vi "Create from SSH.vi"(8 "Error In":errorcluster, 11 "SSH":refnum<class "SSH.lvclass">) -> (0 "Error Out":errorcluster, 3 "Identity":refnum<class "Agent Identity.lvclass">)   [LabVIEW 2018, in "Toolkit.lvlib" / "Agent Identity.lvclass"]
uses:
  Agent Identity.lvclass
  SSH/SSH.lvclass
  SSH/SSH.lvclass/SSH.ctl
  Agent Identity.lvclass/Agent Identity.ctl
  Toolkit.lvlib
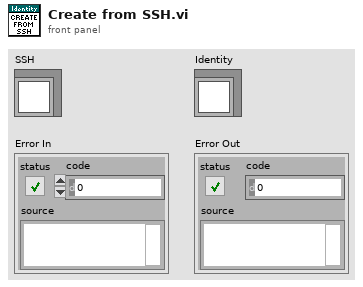
[diagram p1: front panel]
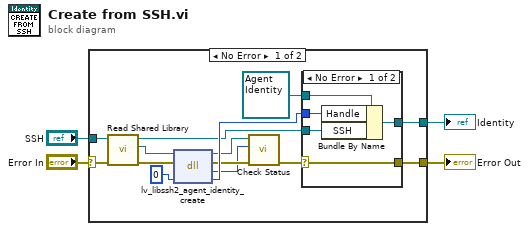
[diagram p0: block diagram]
diagram:
  n1 = case shown="No Error" "Error In" {
    selector: "Error In" -> [w6 w26]
    tunnel: [w9 w26] -> w3
    tunnel: "SSH" -> [w7 _]
    tunnel: [w18 _] -> w1
    frame No Error {
      n2 = call "Read Shared Library.vi"("Error In"=w6, "SSH In"=w7) -> ("Error Out"=w17:errorcluster, "lv-libssh2 Shared Library"=w16:path, "SSH Out"=w8:refnum<class "SSH.lvclass">)  [unwired: 7 in]
      n3 = dll-call lib="libssh2lv.*" fn="lv_libssh2_agent_identity_create"(path in=w16, error in=w17, "handle"=u64 0) -> (path out=w11:path, error out=w13:errorcluster, "status"=w12:i32, "handle"=w14:u64)  [unwired: 1 in]
      n4 = call "Check Status.vi"("Error In"=w13, "Status"=w12, "lv-libssh2 Shared Library In"=w11) -> ("Error Out"=w10:errorcluster)  [unwired: 7 in, 1 out]
      n5 = case shown="No Error" w10 {
        selector: w10 -> [w22 w25]
        tunnel: [w19 w24] -> w18
        tunnel: w14 -> [w23 _]
        tunnel: [w22 w25] -> w9
        tunnel: w8 -> [w21 _]
        tunnel: refnum<class "Agent Identity.lvclass"> refnum ("Toolkit.lvlib:Agent Identity.lvclass") -> [w20 w24]
        frame No Error {
          n6 = Bundle By Name(cluster=w20, "Handle"=w23, "SSH"=w21) -> (w19:refnum<class "Agent Identity.lvclass">)
        }
        frame Error {
        }
      }
    }
    frame Error {
    }
  }
  "Error Out" <- w3
  "Identity" <- w1
